vi "AddEdge.vi"(4 "end":i32, 5 "start":i32, 9 "DAG in":refnum<class "DAG.lvclass">) -> (3 "DAG out":refnum<class "DAG.lvclass">)   [LabVIEW 2014, in "DAG.lvclass"]
uses:
  DAG.lvclass
  DAG.lvclass/DAG.ctl
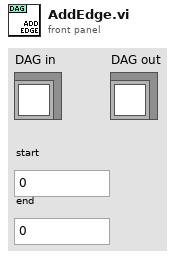
[diagram p1: front panel]
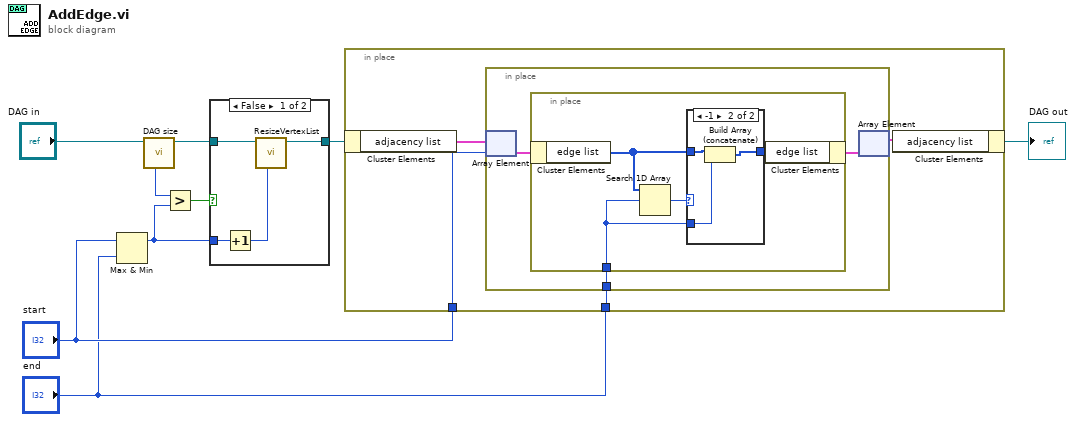
[diagram p0: block diagram]
diagram:
  n1 = Max & Min(x="start", y="end") -> (max(x,y)=w5:i32)  [unwired: 1 out]
  n2 = call "DAG size.vi"("DAG in"="DAG in") -> ("DAG out"=w8:refnum<class "DAG.lvclass">, "vertices"=w7:i32)  [unwired: 6 in, 1 out]
  n3 = Greater?(x=w7, y=w5) -> (0:w6:bool)
  n4 = case shown="False" w6 {
    tunnel: w8 -> [w13 w14]
    tunnel: w5 -> [w12 _]
    tunnel: [w10 w14] -> w4
    frame False {
      n5 = Increment(x=w12) -> (x+1=w11:i32)
      n6 = call "ResizeVertexList.vi"("size"=w11, "DAG in"=w13) -> ("DAG out"=w10:refnum<class "DAG.lvclass">)  [unwired: 7 in]
    }
    frame True {
    }
  }
  n7 = in-place {
    in-place-border: "start" -> [w17]
    in-place-border: "end" -> [w15]
    n8 = in-place-cluster #1(w4) -> ("adjacency list"=w18:cluster{"edge list":i32[]}[])
    n9 = in-place {
      in-place-border: w15 -> [w19]
      n10 = in-place-array #2(w18, w17) -> (w21:cluster{"edge list":i32[]})
      n11 = in-place {
        in-place-border: w19 -> [w22]
        n12 = in-place-cluster #3(w21) -> ("edge list"=w23:i32[])
        n13 = Search 1D Array(1D array=w23, element=w22) -> (index of element=w24:i32)  [unwired: 1 in]
        n14 = case shown="-1" w24 {
          tunnel: [w26 w29] -> w25
          tunnel: w23 -> [w26 w28]
          tunnel: w22 -> [_ w27]
          frame Default {
          }
          frame -1 {
            n15 = Build Array (concatenate)(w28, w27) -> (w29:i32[])
          }
        }
        n16 = in-place-cluster #3("edge list"=w25) -> (w20:cluster{"edge list":i32[]})
      }
      n17 = in-place-array #2(w20) -> (w16:cluster{"edge list":i32[]}[])  [unwired: 1 out]
    }
    n18 = in-place-cluster #1("adjacency list"=w16) -> (→"DAG out":refnum<class "DAG.lvclass">)
  }
